vi "Validate Pulse duration.vi"(1 "Pulse Duration":u32[](array[numeric])) -> (0 "Pulse Duration":u32[](array[numeric]))   [LabVIEW 2019]
panel:
  in  "Pulse Duration":u16
  out "Warning":string
  out "Pulse duration":u16
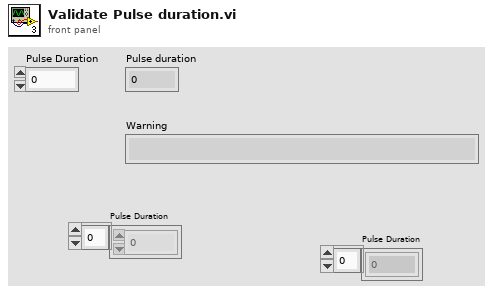
[diagram p1: front panel]
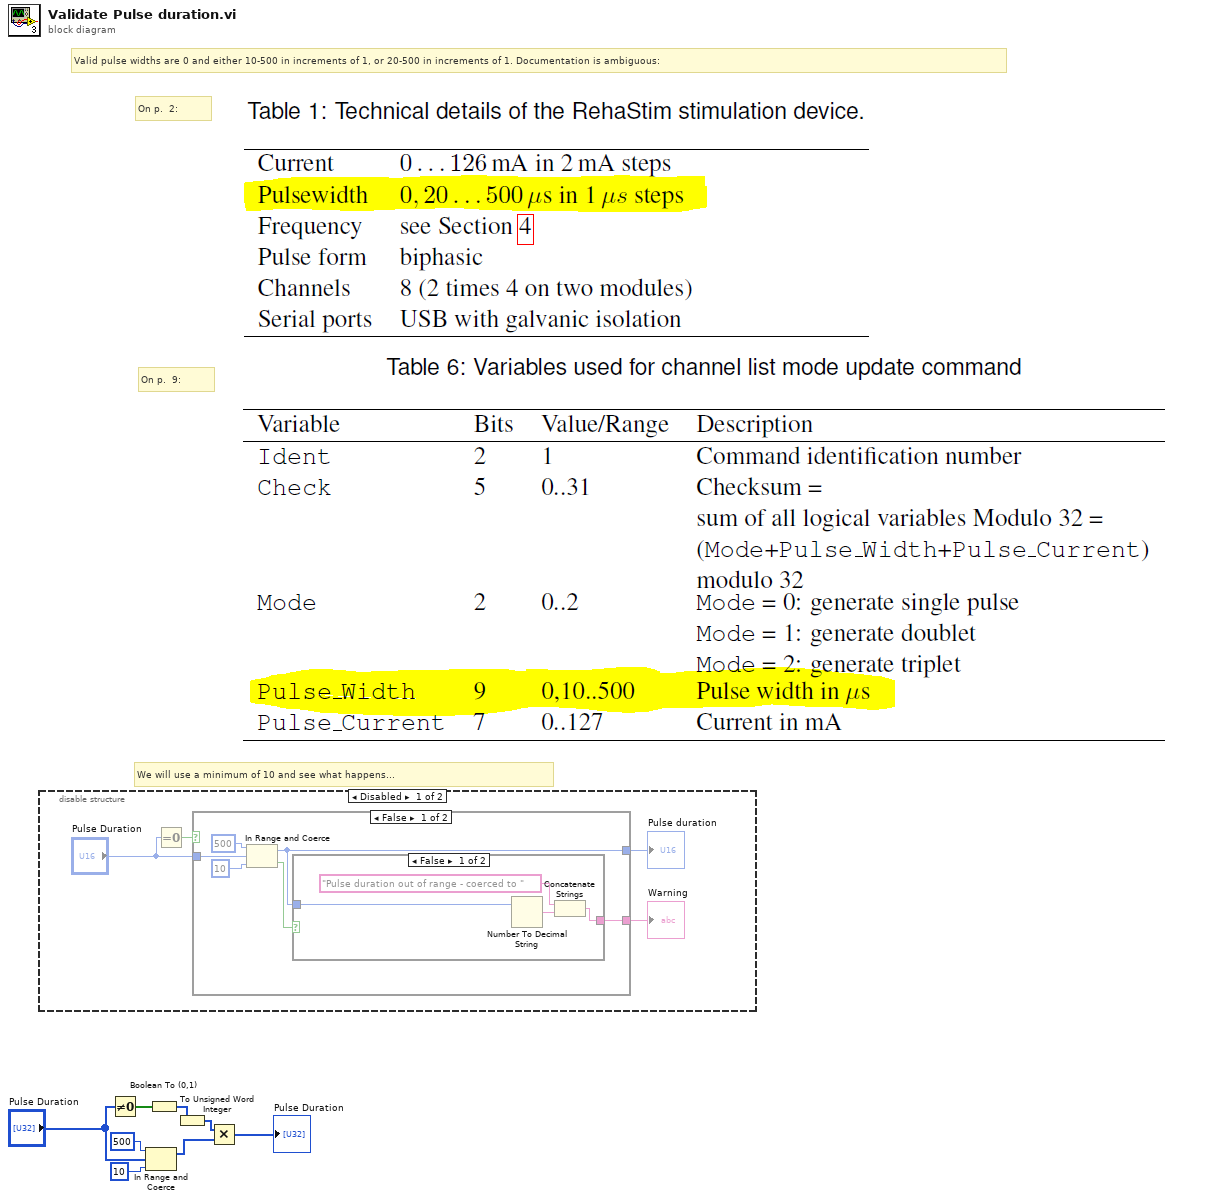
[diagram p0: block diagram]
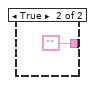
[diagram p2: hidden frame]
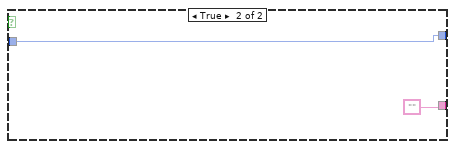
[diagram p3: hidden frame]
diagram:
  # "We will use a minimum of 10 and see what happens..."
  # "On p.  9:"
  # "On p.  2:"
  # "Valid pulse widths are 0 and either 10-500 in increments of 1, or 20-500 in increments of 1. Documentation is ambiguous:"
  n1 = disable-structure shown="Disabled" {
    frame Disabled {
      n2 = Equal To 0?(x="Pulse Duration") -> (x = 0?=w12:bool)
      n3 = case shown="False" w12 {
        tunnel: "Pulse Duration" -> [w17 w25]
        tunnel: [w14 ""] -> w10
        tunnel: [w13 w25] -> w9
        frame False {
          n4 = In Range and Coerce(upper limit=u16 500, x=w17, lower limit=i16 10) -> (coerced(x)=w13:u16, In Range?=w18:bool)
          n5 = case shown="False" w18 {
            tunnel: w13 -> [w19 _]
            tunnel: [w20 ""] -> w14
            frame False {
              n6 = Number To Decimal String(number=w19) -> (decimal integer string=w21:string)  [unwired: 1 in]
              n7 = Concatenate Strings("Pulse duration out of range - coerced to ", w21) -> (w20:string)
            }
            frame True {
            }
          }
        }
        frame True {
        }
      }
      "Pulse duration" <- w9
      "Warning" <- w10
    }
    frame Enabled {
    }
  }
  n8 = Not Equal To 0?(x="Pulse Duration") -> (x != 0?=w8:bool[])
  n9 = In Range and Coerce(upper limit=u16 500, x="Pulse Duration", lower limit=u16 10) -> (coerced(x)=w7:u32[])  [unwired: 1 out]
  n10 = Boolean To (0,1)(Boolean=w8) -> (0, 1=w4:i16[])
  n11 = To Unsigned Word Integer(number=w4) -> (unsigned 16bit integer=w3:u16[])
  n12 = Multiply(x=w3, y=w7) -> (x*y=→"Pulse Duration":u32[])
